vi "Rearrange TDMS Data.vi"(8 "error in (no error)":errorcluster, 9 "TDMS Group Channel Order":T1[](array[typedef]), 10 "Existing TDMS Path":path, 11 "New TDMS Path":path) -> (0 "error out":errorcluster)   [LabVIEW 2015]
doc: "This VI will rearrange the data in a TDMS file based on the <B>TDMS Group Channel Order</B>. Pass the <B>Existing TDMS Path</B> in and then a path for the <B>New TDMS Path</B> to be saved which will contain the same data as the Existing file, but with the order of the groups and channels updated.\n\n-----\nBrian Hoover (Hooovahh)"
uses:
  TDMS Group Information.ctl
  Combine TDMS Files Into One.vi
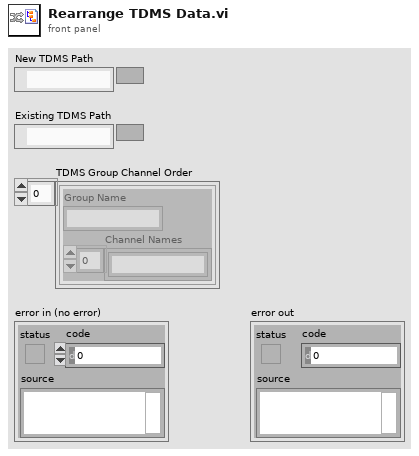
[diagram p1: front panel]
types:
  T1 = typedef "TDMS Group Information.ctl" = cluster{"Group Name":string, "Channel Names":string[]}
  T2 = enum16{"open", "open or create", "create or replace", "create", "open (read-only)"}
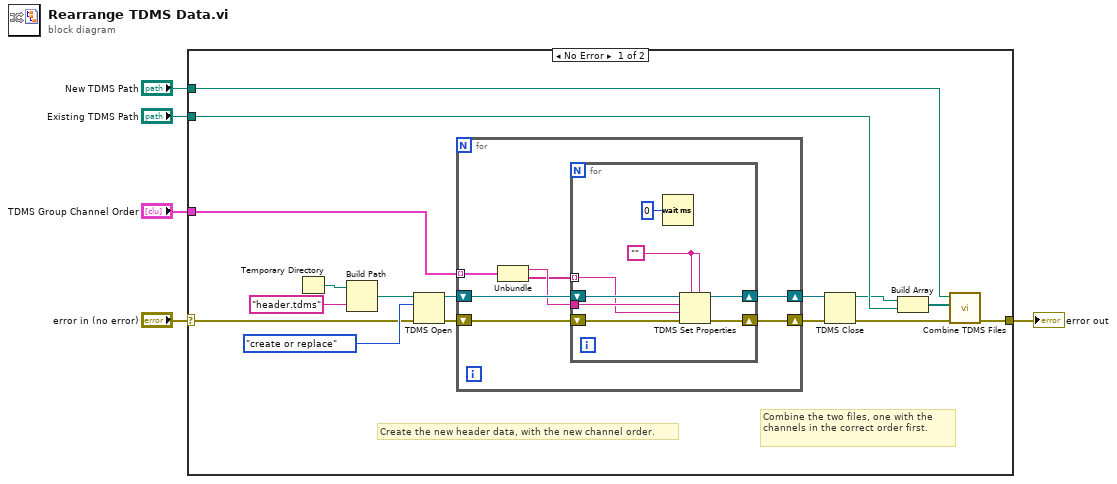
[diagram p0: block diagram]
diagram:
  n1 = case shown="No Error" "error in (no error)" {
    selector: "error in (no error)" -> [w6 w37]
    tunnel: "TDMS Group Channel Order" -> [w21 _]
    tunnel: [w20 w37] -> w4
    tunnel: "New TDMS Path" -> [w19 _]
    tunnel: "Existing TDMS Path" -> [w16 _]
    frame No Error {
      # "Combine the two files, one with the channels in the correct order first."
      # "Create the new header data, with the new channel order."
      n2 = Temporary Directory() -> (w9:path)
      n3 = Build Path(base path=w9, name or relative path="header.tdms") -> (appended path=w7:path)
      n4 = TDMS Open(8:w6, 10:T2."create or replace" ("operation (0:open)"), 11:w7) -> (0:w13:errorcluster, 3:w14:refnum<k34>)  [unwired: 4 in]
      n5 = for {
        shift-right: [w26] -> w11
        shift-left: w14 -> [w28]
        shift-right: [w25] -> w10
        shift-left: w13 -> [w27]
        tunnel: w21 -> [w24] mode=indexing
        n6 = Unbundle(w24) -> ("Group Name"=w23:string, "Channel Names"=w22:string[])
        n7 = for {
          tunnel: w23 -> [w33]
          shift-right: [w34] -> w26
          shift-left: w28 -> [w36]
          shift-right: [w31] -> w25
          shift-left: w27 -> [w35]
          tunnel: w22 -> [w32] mode=indexing
          w30 = ""
          n8 = Wait (ms)(milliseconds to wait=u32 0) -> ()  [unwired: 1 out]
          n9 = TDMS Set Properties(5:w30, 7:w30, 8:w35, 9:w32, 10:w33, 11:w36) -> (0:w31:errorcluster, 3:w34:refnum<k34>)  [unwired: 2 out]
        }
      }
      n10 = TDMS Close(8:w10, 11:w11) -> (0:w18:errorcluster, 3:w15:path)
      n11 = Build Array(w15, w16) -> (w17:path[])
      n12 = call-poly "Combine TDMS Files.vi"("error in (no error)"=w18, "TDMS Files"=w17, "Combined TDMS Path"=w19) -> ("error out"=w20:errorcluster)  [unwired: 7 in, 1 out]
    }
    frame Error {
    }
  }
  "error out" <- w4
